vi "iterate_VanDerPauw.vi"(8 "thickness /cm":dbl, 9 "Rb":dbl=10.0, 10 "Ra":dbl=10.0, 11 "Error Limit":dbl=0.0005) -> (0 "iterations":i32=2, 2 "rho /Ohm cm":dbl, 3 "R sheet":dbl=45.323601418271934 format="%_8g")   [LabVIEW 2018]
doc: "Use this template to build a standard state machine design pattern. Each state executes code and determines which state to transition to. Contrast this design pattern with the User Interface Event Handler pattern, in which code executes in response to user actions. Contrast this design pattern also with the Queued Message Handler pattern, in which each message handling code can queue zero or more new messages."
panel:
  # "Van Der Pauw Equation Solver"
  # "Input to Equation"
  # "Output from Equation"
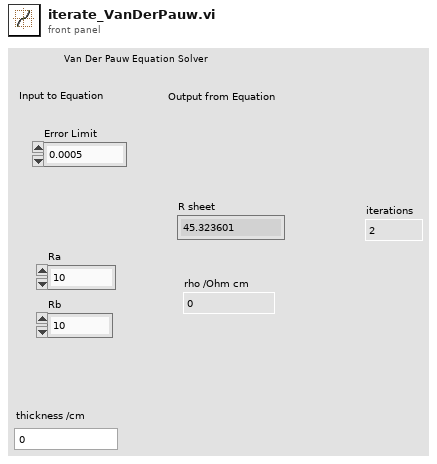
[diagram p1: front panel]
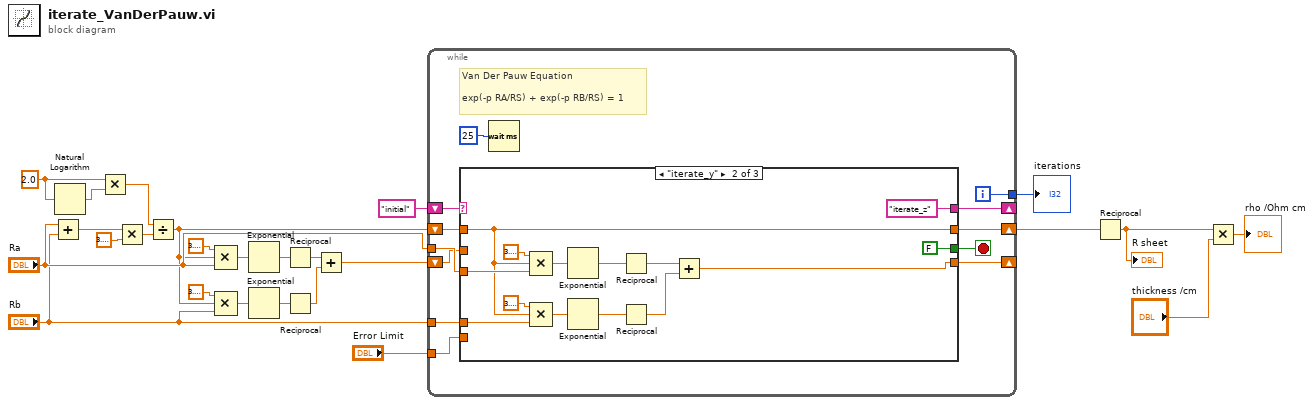
[diagram p0: block diagram]
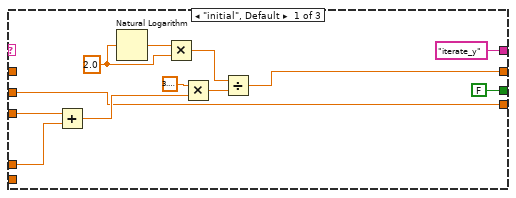
[diagram p2: hidden frame]
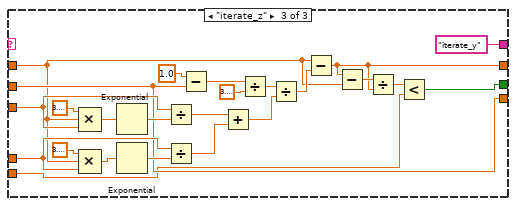
[diagram p3: hidden frame]
diagram:
  w22 = 2.0 ("x")
  n1 = Add(x="Ra", y="Rb") -> (x+y=w18:dbl)
  n2 = Natural Logarithm(1:w22) -> (0:w21:dbl)
  n3 = Multiply(x=w22, y=w21) -> (x*y=w20:dbl)
  n4 = Multiply(x=w18, y=3.141592653589793) -> (x*y=w17:dbl)
  n5 = Divide(x=w20, y=w17) -> (x/y=w9:dbl)
  n6 = Compound Arithmetic op=MULTIPLY(3.141592653589793, w9, "Ra") -> (w16:dbl)
  n7 = Compound Arithmetic op=MULTIPLY(3.141592653589793, w9, "Rb") -> (w10:dbl)
  n8 = Exponential(1:w16) -> (0:w13:dbl)
  n9 = Exponential(1:w10) -> (0:w12:dbl)
  n10 = Reciprocal(x=w13) -> (1/x=w7:dbl)
  n11 = Reciprocal(x=w12) -> (1/x=w6:dbl)
  n12 = Add(x=w7, y=w6) -> (x+y=w5:dbl)
  n13 = while {
    shift-right: [w36] -> _
    shift-left: "initial" -> [w37]
    shift-right: [w30] -> _
    shift-left: w5 -> [w29]
    shift-right: [w32] -> w24
    shift-left: w9 -> [w31]
    tunnel: "Ra" -> [w34]
    tunnel: "Rb" -> [w33]
    tunnel: "Error Limit" -> [w28]
    tunnel: [w26] -> w4
    i -> [w26]
    stop <- w27 stop-if-true
    # "Van Der Pauw Equation\n\nexp(-p RA/RS) + exp(-p RB/RS) = 1"
    n14 = case shown="\"iterate_y\"" w37 {
      tunnel: ["iterate_y" "iterate_z" "iterate_y"] -> w36
      tunnel: w34 -> [w49 w55 w80]
      tunnel: w33 -> [w48 w54 w81]
      tunnel: [w41 w53 w68] -> w32
      tunnel: w31 -> [_ w53 w70]
      tunnel: [w40 w52 w71] -> w30
      tunnel: w29 -> [w40 _ w71]
      tunnel: w28 -> [_ _ w66]
      tunnel: [FALSE FALSE w65] -> w27
      frame "initial", Default {
        w44 = 2.0 ("x")
        n15 = Add(x=w49, y=w48) -> (x+y=w47:dbl)
        n16 = Natural Logarithm(1:w44) -> (0:w45:dbl)
        n17 = Multiply(x=w45, y=w44) -> (x*y=w43:dbl)
        n18 = Multiply(x=3.141592653589793, y=w47) -> (x*y=w42:dbl)
        n19 = Divide(x=w43, y=w42) -> (x/y=w41:dbl)
      }
      frame "iterate_y" {
        n20 = Compound Arithmetic op=MULTIPLY(3.141592653589793, w53, w55) -> (w59:dbl)
        n21 = Compound Arithmetic op=MULTIPLY(3.141592653589793, w53, w54) -> (w62:dbl)
        n22 = Exponential(1:w59) -> (0:w60:dbl)
        n23 = Exponential(1:w62) -> (0:w61:dbl)
        n24 = Reciprocal(x=w60) -> (1/x=w57:dbl)
        n25 = Reciprocal(x=w61) -> (1/x=w56:dbl)
        n26 = Add(x=w57, y=w56) -> (x+y=w52:dbl)
      }
      frame "iterate_z" {
        n27 = Compound Arithmetic op=MULTIPLY(3.141592653589793, w70, w80) -> (w85:dbl)
        n28 = Compound Arithmetic op=MULTIPLY(3.141592653589793, w70, w81) -> (w86:dbl)
        n29 = Exponential(1:w85) -> (0:w83:dbl)
        n30 = Exponential(1:w86) -> (0:w82:dbl)
        n31 = Divide(x=w80, y=w83) -> (x/y=w79:dbl)
        n32 = Divide(x=w81, y=w82) -> (x/y=w78:dbl)
        n33 = Subtract(x=1.0, y=w71) -> (x-y=w76:dbl)
        n34 = Add(x=w79, y=w78) -> (x+y=w73:dbl)
        n35 = Divide(x=w76, y=3.141592653589793) -> (x/y=w74:dbl)
        n36 = Divide(x=w74, y=w73) -> (x/y=w72:dbl)
        n37 = Subtract(x=w70, y=w72) -> (x-y=w68:dbl)
        n38 = Subtract(x=w68, y=w70) -> (x-y=w69:dbl)
        n39 = Divide(x=w69, y=w68) -> (x/y=w67:dbl)
        n40 = Less?(x=w67, y=w66) -> (x < y?=w65:bool)
      }
    }
    n41 = Wait (ms)(milliseconds to wait=u32 25) -> ()  [unwired: 1 out]
  }
  "iterations" <- w4
  n42 = Reciprocal(x=w24) -> (1/x=w3:dbl)
  "R sheet" <- w3
  n43 = Multiply(x=w3, y="thickness /cm") -> (x*y=→"rho /Ohm cm":dbl)
